vi "Pre Launch Init.vi"(11 "Master Controller in":refnum<class "Master Controller.lvclass">) -> (0 "error out":errorcluster, 3 "Master Controller out":refnum<class "Master Controller.lvclass">)   [LabVIEW 2015, in "Master Controller Core.lvlib" / "Master Controller.lvclass"]
doc: "(<B>Filename</B>: Actor Framework.lvlib:Actor.lvclass:Pre Launch Init.vi)\n\nDefines behavior that occurs after the Launch Nested Actor method is invoked but before the actor's Actor Core method begins running.\n\nBy default, this method does nothing. A descendant class may override it to define behavior."
uses:
  Master Controller.lvclass
  Master Controller.lvclass/Master Controller.ctl
  <vilib>/ActorFramework/Actor/Actor.lvclass
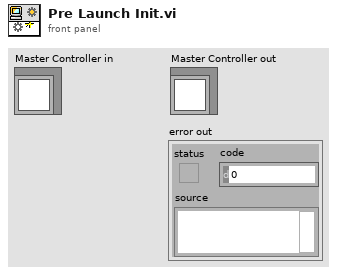
[diagram p1: front panel]
types:
  T1 = typedef "Master Controller Core.lvlib/Master Controller.lvclass/Master Controller notifiers.ctl" = cluster{"SCADA\nstop":refnum<notifier>, "Main Comms\nstop":refnum<notifier>, "Emergency\nComms stop":refnum<notifier>, "Viz Comms\nstop":refnum<notifier>}
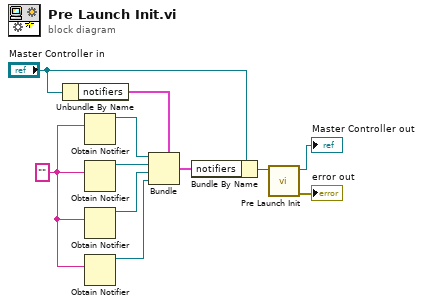
[diagram p0: block diagram]
diagram:
  w4 = "" ("Status Update")
  n1 = Unbundle By Name("Master Controller in") -> ("notifiers"=w9:T1)
  n2 = Obtain Notifier(notification data type=w4) -> (notifier out=w5:refnum<notifier>)  [unwired: 3 in, 2 out]
  n3 = Obtain Notifier(notification data type=w4) -> (notifier out=w3:refnum<notifier>)  [unwired: 3 in, 2 out]
  n4 = Obtain Notifier(notification data type=w4) -> (notifier out=w2:refnum<notifier>)  [unwired: 3 in, 2 out]
  n5 = Obtain Notifier(notification data type=w4) -> (notifier out=w1:refnum<notifier>)  [unwired: 3 in, 2 out]
  n6 = Bundle(cluster=w9, "SCADA\nstop"=w5, "Main Comms\nstop"=w3, "Emergency\nComms stop"=w2, "Viz Comms\nstop"=w1) -> (w7:T1)
  n7 = Bundle By Name(cluster="Master Controller in", "notifiers"=w7) -> (w6:refnum<class "Master Controller.lvclass">)
  n8 = call-parent "Pre Launch Init.vi"("Actor in"=w6) -> ("error out"=→"error out":errorcluster, "Actor out"=→"Master Controller out":refnum<class "Master Controller.lvclass">)  [unwired: 9 in]
